vi "Intan_mainControlPanel_128ch.vi"() -> ()   [LabVIEW 2020]
panel:
  in  "Experiment Duration (hr)":dbl=1.0
  out "FileSize(MB)":i16
  out "ADC calib":bool
  in  "Config Hardware Filter":bool=TRUE
  in  "ConfigReg [0:7, aPwr]":bool=TRUE
  in  "R_L source":u8(ring)=1 items=["ON-chip", "OFF-chip"]
  in  "Lower cutoff":u8(ring)=12 items=["10 Hz", "7.5 Hz", "5.0 Hz", "3.0 Hz", "2.5 Hz", "2.0 Hz", "1.5 Hz", "1.0 Hz", "0.75 Hz", "0.5 Hz", "0.3 Hz", "0.25 Hz", "0.10 Hz"]
  in  "Upper cutoff":u8(ring)=12 items=["5.0 kHz", "3.0 kHz", "2.5 kHz", "2.0 kHz", "1.5 kHz", "1.0 kHz", "750 Hz", "500 Hz", "300 Hz", "250 Hz", "200 Hz", "150 Hz", "100 Hz"]
  out "NumMaxStreamingChans":u16
  out "DT samp (us)":dbl
  out "ADC fs (Hz)":dbl
  in  "Desired Fs (Hz)":u16=100
  in  "Save to SD card":bool=TRUE
  in  "SD File Name Suffix\n (2 digits)":string="51"
  out "Serial Port Type":string
  in  "VISA resource name":refnum<visa-resource-name>="COM33"
  in  "Start Data Stream":bool
  out "HeaderFilePath":path
  in  "Save Display Data":bool
  out "Config Result":string
  out "Teensy response":string
  out "Raw data file path":path
  in  "Save Raw Data":bool
  # "Intan-Teensy Bioelectric Module: \nconfigure hardware and serial port \nAmbulatory 128 chan"
  # "Configure all settings, then click run arrow.\n\nWhen config is complete, click the purple\nbutton to start data stream.\n\nSeparate VI will pop open to display signals"
  # "Serial Streaming"
  # "Intan Amp Config"
  # "Hardware Filter Settings"
  # "ADC Sampling"
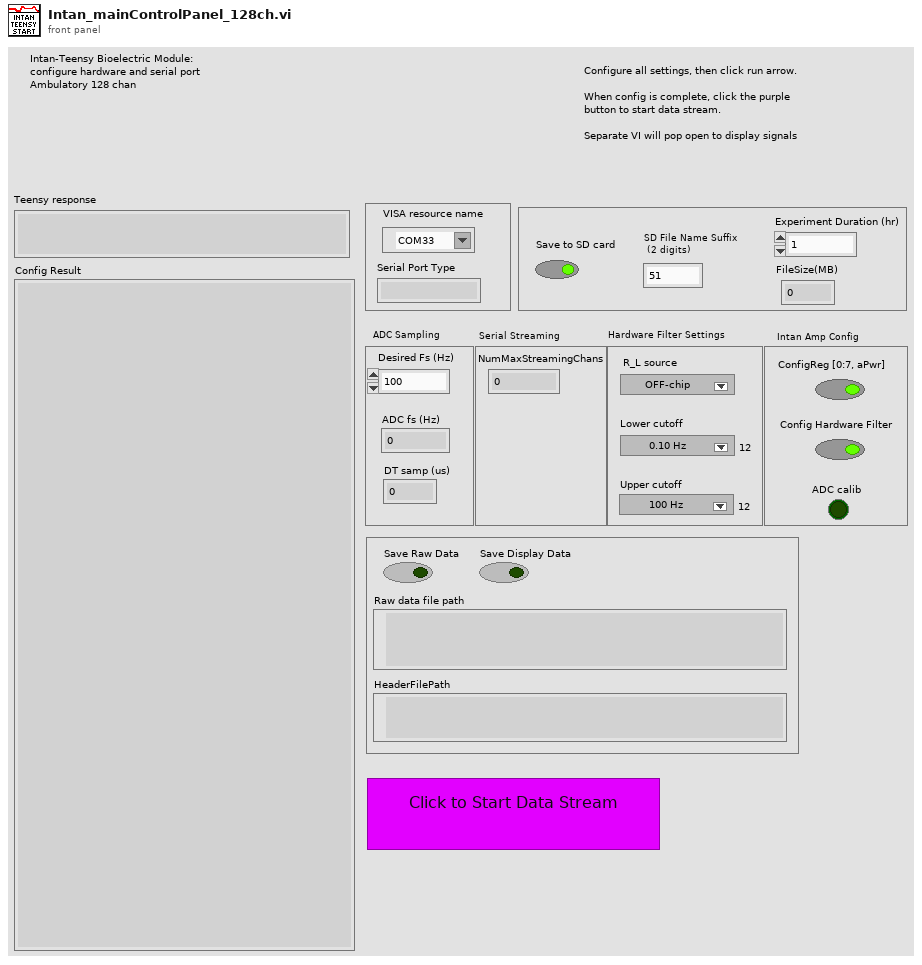
[diagram p1: front panel]
types:
  T1 = enum8{"Enabled", "Disabled", "Disabled and Grayed Out"}
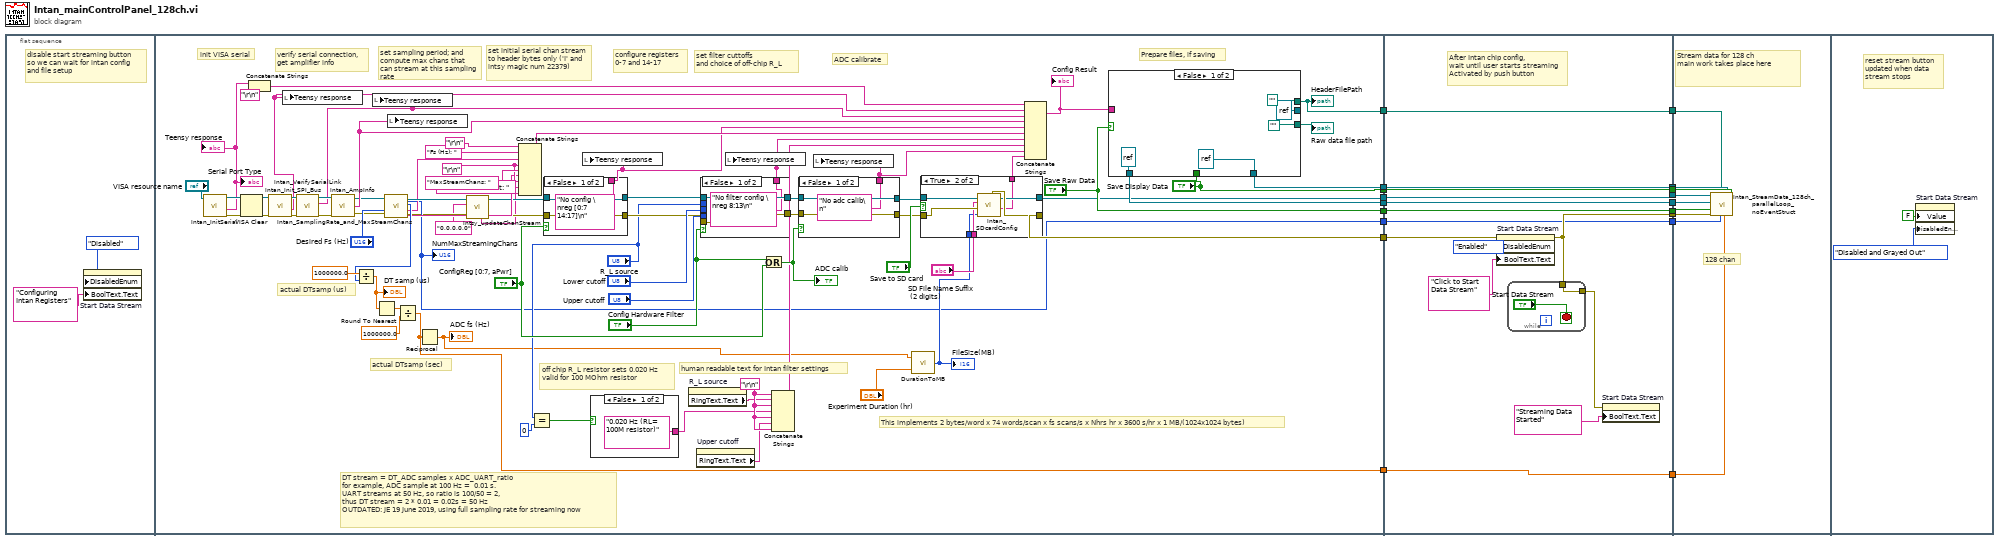
[diagram p0: block diagram]
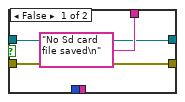
[diagram p2: hidden frame]
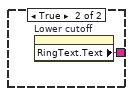
[diagram p3: hidden frame]
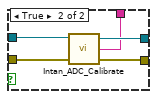
[diagram p4: hidden frame]
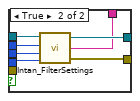
[diagram p5: hidden frame]
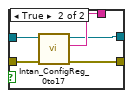
[diagram p6: hidden frame]
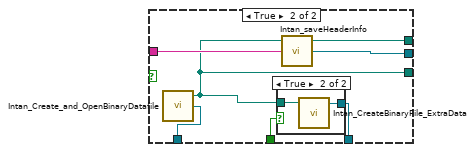
[diagram p7: hidden frame]
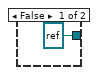
[diagram p8: hidden frame]
diagram:
  n1 = flat-sequence {
    tunnel: [w91] -> w12
    tunnel: [w31] -> w11
    tunnel: [w81] -> w10
    tunnel: ["Save Raw Data"] -> w9
    tunnel: ["Save Display Data"] -> w8
    tunnel: [w42] -> w7
    tunnel: [w64] -> w4
    tunnel: [w40] -> w3
    tunnel: [w27] -> w2
    tunnel: [w158] -> w18
    tunnel: [w164] -> w17
    tunnel: [w163] -> w16
    tunnel: [w162] -> w15
    tunnel: [w161] -> w14
    tunnel: [w160] -> w13
    tunnel: w8 -> [w160]
    tunnel: w9 -> [w161]
    tunnel: w10 -> [w162]
    tunnel: w11 -> [w163]
    tunnel: w12 -> [w164]
    tunnel: w7 -> [w157]
    tunnel: [w156] -> w6
    tunnel: [w155] -> w5
    tunnel: w4 -> [w155]
    tunnel: w3 -> [w156]
    tunnel: w2 -> [w151]
    tunnel: [w151] -> w1
    tunnel: w18 -> [w172]
    tunnel: w17 -> [w170]
    tunnel: w16 -> [w175]
    tunnel: w15 -> [w173]
    tunnel: w14 -> [w171]
    tunnel: w13 -> [w174]
    tunnel: w6 -> [w169]
    tunnel: w5 -> [w168]
    tunnel: w1 -> [w167]
    frame #0 {
      # "disable start streaming button\nso we can wait for intan config\nand file setup"
      n2 = property on="Start Data Stream" class="Bool (strict)"("DisabledEnum"=T1."Disabled" ("Disabled"), "BoolText.Text"="Configuring Intan Registers" ("Boolean Text.Text")) -> ()  [unwired: 2 in, 2 out]
    }
    frame #1 {
      w59 = "\r\n"
      w36 = "\r\n"
      # "set initial serial chan stream to header bytes only ('I' and intsy magic num 22379)"
      # "This implements 2 bytes/word x 74 words/scan x fs scans/s x Nhrs hr x 3600 s/hr x 1 MB/(1024x1024 bytes)"
      # "DT stream = DT_ADC samples x ADC_UART_ratio\nfor example, ADC sample at 100 Hz =  0.01 s.\nUART streams at 50 Hz, so ratio is 100/50 = 2,\nthus DT stream = 2 * 0.01 = 0.02s = 50 Hz\nOUTDATED: JE 19 June 2019, using full sampling rate for streaming now"
      # "off chip R_L resistor sets 0.020 Hz \nvalid for 100 MOhm resistor"
      # "human readable text for Intan filter settings"
      # "Prepare files, if saving"
      # "ADC calibrate"
      # "set filter cuttoffs \nand choice of off-chip R_L"
      # "configure registers\n0-7 and 14-17"
      # "set sampling period; and compute max chans that can stream at this sampling rate"
      # "verify serial connection,\nget amplifier info"
      # "init VISA serial"
      # "actual DTsamp (sec)"
      # "actual DTsamp (us)"
      n3 = call "Intan_InitSerial.vi"("VISA resource name"="VISA resource name") -> ("VISA resource name out"=w63:refnum<visa-resource-name>, "Text response"=w61:string, "error out"=w90:errorcluster)  [unwired: 3 in]
      "Teensy response" <- w61
      "Serial Port Type" <- w61
      n4 = VISA Clear(VISA resource name=w63, error in (no error)=w90) -> (VISA resource name out=w50:refnum<visa-resource-name>, error out=w49:errorcluster)
      n5 = Concatenate Strings(w61, "\r\n") -> (w46:string)
      n6 = call "Intan_Init_SPI_Bus.vi"("error in"=w49, "VISA resource name"=w50) -> ("error out"=w48:errorcluster, "SPIinitResponses"=w45:string, "VISA resource name out"=w47:refnum<visa-resource-name>)  [unwired: 3 in]
      n7 = local write "Teensy response"(w45) -> ()
      n8 = call "Intan_VerifySerialLink.vi"("error in"=w48, "VISA resource name"=w47) -> ("error out"=w92:errorcluster, "verifySpiResponse"=w88:string, "VISA resource name out"=w93:refnum<visa-resource-name>)  [unwired: 7 in]
      n9 = call "Intan_AmpInfo.vi"("error in"=w92, "VISA resource name"=w93) -> ("error out"=w77:errorcluster, "ampInfoTextResponse"=w89:string, "VISA resource name out"=w78:refnum<visa-resource-name>)  [unwired: 1 in]
      n10 = local write "Teensy response"(w88) -> ()
      n11 = call "Intan_SamplingRate_and_MaxStreamChans.vi"("VISA resource name"=w78, "error in"=w77, "Desired Fs (Hz)"="Desired Fs (Hz)") -> ("VISA resource name out"=w76:refnum<visa-resource-name>, "error out"=w25:errorcluster, "NstreamChansmax"=w27:i32, "FS actual (Hz)"=w30:i32, "Actual Sampling Frequency (Hz)"=w29:string, "NchansmaxStr"=w28:string)  [unwired: 1 in]
      "NumMaxStreamingChans" <- w27
      n12 = Divide(x=1000000.0, y=w30) -> (x/y=w35:dbl)
      "DT samp (us)" <- w35
      n13 = Round To Nearest(number=w35) -> (nearest integer value=w84:dbl)
      n14 = local write "Teensy response"(w89) -> ()
      n15 = Divide(x=w84, y=1000000.0 ("x")) -> (x/y=w31:dbl)
      n16 = Reciprocal(x=w31) -> (1/x=w33:dbl)
      "ADC fs (Hz)" <- w33
      n17 = call "Intsy_updateChanStream.vi"("error in (no error)"=w25, "ChanSelString"="0,0,0,0,0", "VISA resource name"=w76) -> ("error out"=w24:errorcluster, "VISA resource name out"=w26:refnum<visa-resource-name>, "NStreamChansString"=w21:string)  [unwired: 5 in, 1 out]
      n18 = Concatenate Strings("\r\n", "Fs (Hz): " ("string"), w29, w36, "MaxStreamChans: " ("string"), w28, w36, "NchansStreamInit: " ("string"), w21) -> (w87:string)
      n19 = Equal?(x="R_L source", y=u8 0) -> (x = y?=w54:bool)
      n20 = case shown="False" "ConfigReg [0:7, aPwr]" {
        tunnel: w26 -> [w129 w135]
        tunnel: w24 -> [w128 w134]
        tunnel: ["No config \nreg [0:7 14:17]\n" ("Text response") w133] -> w75
        tunnel: [w129 w132] -> w72
        tunnel: [w128 w131] -> w71
        frame False {
        }
        frame True {
          n21 = call "Intan_ConfigReg_0to17.vi"("error in"=w134, "VISA resource name"=w135) -> ("error out"=w131:errorcluster, "configspi0"=w133:string, "VISA resource name out"=w132:refnum<visa-resource-name>)  [unwired: 7 in]
        }
      }
      n22 = local write "Teensy response"(w75) -> ()
      n23 = case shown="False" w54 {
        tunnel: ["0.020 Hz (RL= 100M resistor)" ("string") w108] -> w52
        frame False {
        }
        frame True {
          n24 = property on="Lower cutoff" class="Ring (strict)"() -> ("RingText.Text"=w108:string)  [unwired: 2 in, 2 out]
        }
      }
      n25 = property on="R_L source" class="Ring (strict)"() -> ("RingText.Text"=w57:string)  [unwired: 2 in, 2 out]
      n26 = property on="Upper cutoff" class="Ring (strict)"() -> ("RingText.Text"=w58:string)  [unwired: 2 in, 2 out]
      n27 = case shown="False" "Config Hardware Filter" {
        tunnel: "R_L source" -> [_ w127]
        tunnel: "Lower cutoff" -> [_ w126]
        tunnel: "Upper cutoff" -> [_ w125]
        tunnel: w72 -> [w119 w124]
        tunnel: w71 -> [w118 w123]
        tunnel: [w119 w122] -> w70
        tunnel: [w118 w121] -> w69
        tunnel: ["No filter config \nreg 8:13\n" ("Text response") w120] -> w68
        frame False {
        }
        frame True {
          n28 = call "Intan_FilterSettings.vi"("VISA resource name"=w124, "R_L source"=w127, "Lower cutoff"=w126, "Upper cutoff"=w125, "error in"=w123) -> ("VISA resource name out"=w122:refnum<visa-resource-name>, "Text response spi0"=w120:string, "error out"=w121:errorcluster)
        }
      }
      n29 = local write "Teensy response"(w68) -> ()
      n30 = Or(x="Config Hardware Filter", y="ConfigReg [0:7, aPwr]") -> (x .or. y?=w67:bool)
      "ADC calib" <- w67
      n31 = Concatenate Strings(w59, w57, w59, w52, w59, w58, w59) -> (w55:string)
      n32 = case shown="False" w67 {
        tunnel: w70 -> [w111 w116]
        tunnel: w69 -> [w110 w115]
        tunnel: [w110 w114] -> w41
        tunnel: [w111 w113] -> w39
        tunnel: ["No adc calib\n" ("Text response") w112] -> w56
        frame False {
        }
        frame True {
          n33 = call "Intan_ADC_Calibrate.vi"("error in"=w115, "VISA resource name"=w116) -> ("error out"=w114:errorcluster, "Text response"=w112:string, "VISA resource name out"=w113:refnum<visa-resource-name>)  [unwired: 1 in]
        }
      }
      n34 = local write "Teensy response"(w56) -> ()
      n35 = call "DurationToMB.vi"("Experiment Duration (hr)"="Experiment Duration (hr)", "fs (hz)"=w33) -> ("FileSize(MB)"=w34:i16)
      "FileSize(MB)" <- w34
      n36 = case shown="True" "Save to SD card" {
        tunnel: ["No Sd card file saved\n" ("Text response") w100] -> w43
        tunnel: [w97 w106] -> w42
        tunnel: w41 -> [w97 w105]
        tunnel: w39 -> [w98 w104]
        tunnel: [w98 w103] -> w40
        tunnel: "SD File Name Suffix\n (2 digits)" -> [_ w102]
        tunnel: w34 -> [_ w101]
        frame False {
        }
        frame True {
          n37 = call "Intan_SDcardConfig.vi"("VISA resource name"=w104, "SdFilename"=w102, "error in"=w105, "FileSize(MB)"=w101) -> ("error out"=w106:errorcluster, "VISA resource name out"=w103:refnum<visa-resource-name>, "SDCardResultStr"=w100:string)  [unwired: 3 out]
        }
      }
      n38 = Concatenate Strings(w46, w45, w88, w89, w75, w87, w68, w55, w56, w43) -> (w82:string)
      "Config Result" <- w82
      n39 = case shown="False" "Save Raw Data" {
        tunnel: [refnum<file> refnum ("refnum out") w147] -> w91
        tunnel: w82 -> [_ w146]
        tunnel: [refnum<file> refnum ("refnum out") w145] -> w81
        tunnel: "Save Display Data" -> [_ w144]
        tunnel: [path "" w143] -> w64
        tunnel: [path "" w142] -> w73
        tunnel: [refnum<file> refnum ("hdr_file_ref_num_out") w141] -> _
        frame False {
        }
        frame True {
          n40 = call "Intan_Create_and_OpenBinaryDatafile.vi"() -> ("file path"=w142:path, "refnum out"=w147:refnum<file>)  [unwired: 2 in, 1 out]
          n41 = case shown="True" w144 {
            tunnel: w142 -> [_ w150]
            tunnel: [refnum<file> refnum ("refnum out") w149] -> w145
            frame False {
            }
            frame True {
              n42 = call "Intan_CreateBinaryFile_ExtraData.vi"("DataFilePath"=w150) -> ("refnum out"=w149:refnum<file>)  [unwired: 3 in, 1 out]
            }
          }
          n43 = call "Intan_saveHeaderInfo.vi"("header text"=w146, "DataFilePath"=w142) -> ("hdr_file_ref_num_out"=w141:refnum<file>, "HeaderFilePath"=w143:path)  [unwired: 1 in, 1 out]
        }
      }
      "HeaderFilePath" <- w64
      "Raw data file path" <- w73
    }
    frame #2 {
      # "After Intan chip config,\nwait until user starts streaming\nActivated by push button"
      n44 = property on="Start Data Stream" class="Bool (strict)"(error in=w157, "DisabledEnum"=T1."Enabled" ("Disabled"), "BoolText.Text"="Click to Start Data Stream" ("Boolean Text.Text")) -> (error out=w158:errorcluster)  [unwired: 1 in, 1 out]
      n45 = while {
        tunnel: w158 -> [w165]
        tunnel: [w165] -> w153
        stop <- "Start Data Stream" stop-if-true
      }
      n46 = property on="Start Data Stream" class="Bool (strict)"(error in=w153, "BoolText.Text"="Streaming Data Started" ("Boolean Text.Text")) -> ()  [unwired: 1 in, 2 out]
    }
    frame #3 {
      # "128 chan"
      # "Stream data for 128 ch\nmain work takes place here"
      n47 = call "Intan_StreamData_128ch_parallelLoop_noEventStruct.vi"("VISA resource name"=w169, "refnum in"=w170, "Save Binary Data"=w171, "error in"=w172, "hdr fpath"=w168, "MaxStreamChans"=w167, "DT_scale (sec)"=w175, "aux file ref num"=w173, "save aux file"=w174) -> ()  [unwired: 7 in, 4 out]
    }
    frame #4 {
      # "reset stream button \nupdated when data\nstream stops"
      n48 = property on="Start Data Stream" class="Bool (strict)"("Value"=FALSE ("Start Data Stream"), "DisabledEnum"=T1."Disabled and Grayed Out" ("Disabled")) -> ()  [unwired: 2 in, 2 out]
    }
  }
